vi "ShowSettingsDialog.vi"(10 "IMAQ Refnum in":refnum<k11>, 11 "Camera (in)":T1={"Framerate (Hz)"=100, "Exposure time (us)"=100, "Image size"={"Width"=1280, "Height"=1024}, "Number of buffers"=30}) -> (3 "Camera (out)":T1={"Framerate (Hz)"=100, "Exposure time (us)"=100, "Image size"={"Width"=1280, "Height"=1024}, "Number of buffers"=30})   [LabVIEW 2011]
uses:
  Main/Camera/GenericCameraConfigType.ctl
  Global_GenericIMAQCamera_HardwareConfig.vi
panel:
  in  "Set offsets to center frame":bool
  in  "Send serial cmd":bool
  out "Serial output":string
  in  "Serial input":string
  in  "Get current":bool
  in  "Camera":T1={"Framerate (Hz)"=100, "Exposure time (us)"=100, "Image size"={"Width"=1280, "Height"=1024}, "Number of buffers"=30}
  in  "Cancel":bool
  in  "Save":bool
  # "Dalsa Falcon2: Width needs to be a multiple of 128."
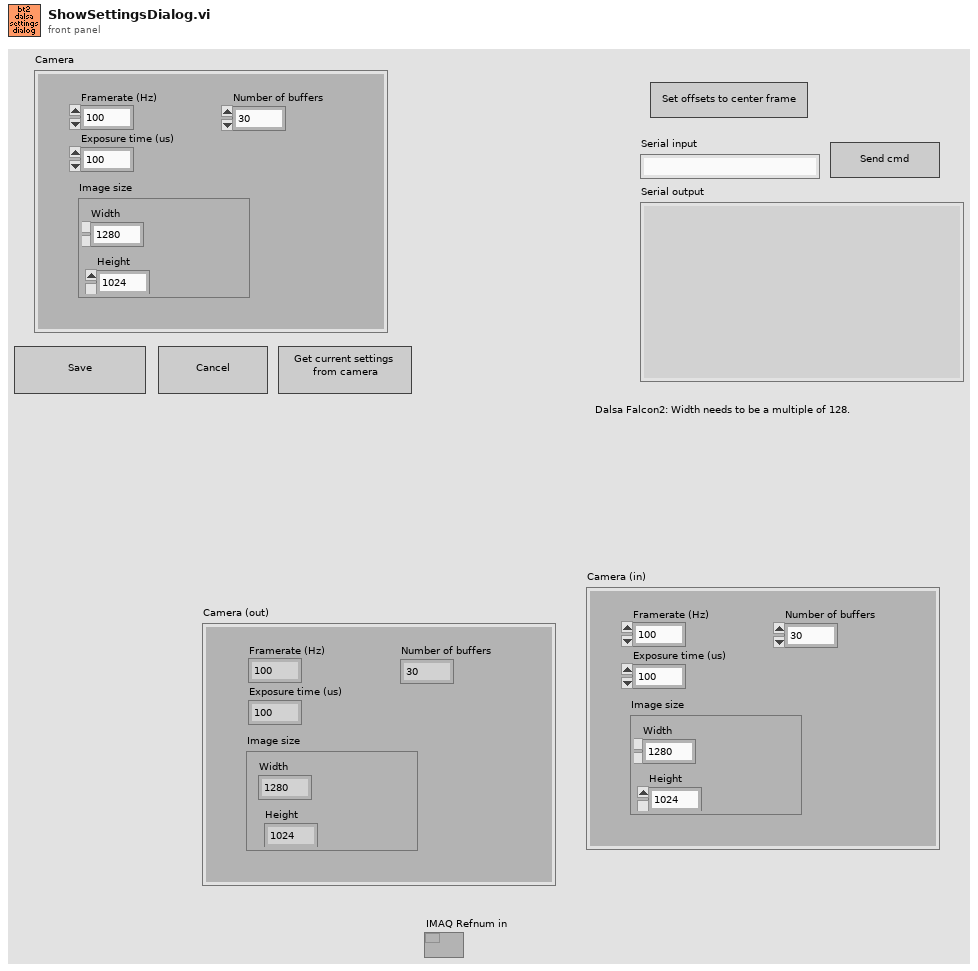
[diagram p1: front panel]
types:
  T1 = typedef "GenericCameraConfigType.ctl" = cluster{"Framerate (Hz)":i32, "Exposure time (us)":i32, "Image size":cluster{"Width":i32, "Height":i32}, "Number of buffers":i32}
  T2 = typedef "GenericIMAQHardwareConfig.ctl" = cluster{"Use serial commands directly":bool, "Frame rate set cmd":string, "Exposure time set cmd":string, "Frame rate get cmd":string, "Exposure time get cmd":string, "IMAQ Identifier":string, "Serial return skip chars":i32, "Set width/height":string, "Set offset xy":string, "Get width":string, "Get height":string, "Get offset X":string, "Get offset Y":string, "Full frame size":cluster{"width":i32, "height":i32}}
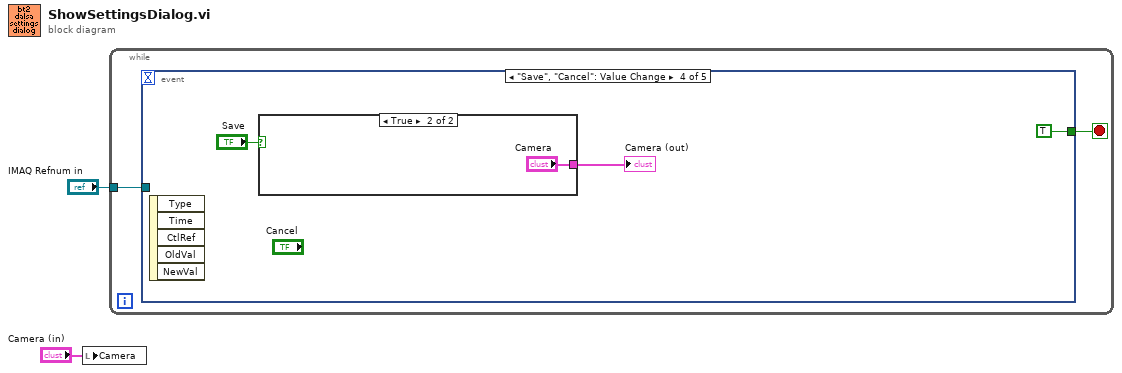
[diagram p0: block diagram]
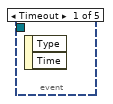
[diagram p2: hidden frame]
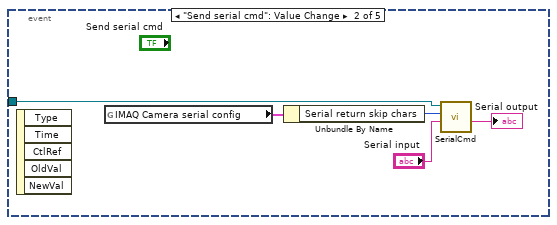
[diagram p3: hidden frame]
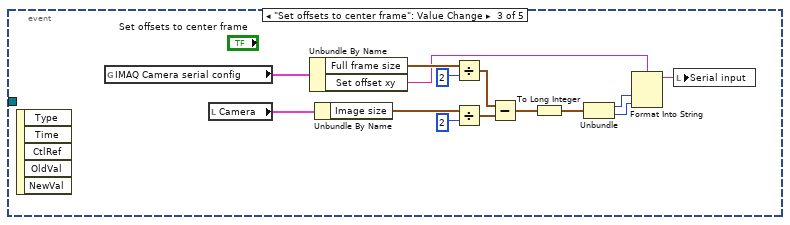
[diagram p4: hidden frame]
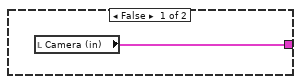
[diagram p5: hidden frame]
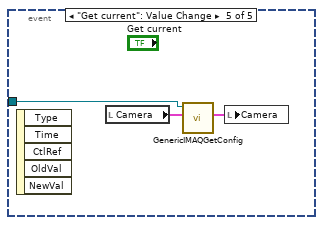
[diagram p6: hidden frame]
diagram:
  n1 = local write "Camera"("Camera (in)") -> ()
  n2 = while {
    tunnel: "IMAQ Refnum in" -> [w3]
    stop <- w4 stop-if-true
    n3 = event shown="[3] \"Save\", \"Cancel\": Value Change" {
      selector: _ -> [_ _ _ _ _]
      dyn-events: _ -> [_ _ _ _ _]
      timeout: _ -> [_ _ _ _ _]
      tunnel: [_ _ _ TRUE _] -> w4
      tunnel: w3 -> [_ w9 _ _ w31]
      event Timeout {
        n4 = event-data() -> ()  [unwired: 1 in, 2 out]
      }
      event "Send serial cmd": Value Change {
        n5 = event-data() -> ()  [unwired: 1 in, 5 out]
        n6 = global read "Global_GenericIMAQCamera_HardwareConfig.vi" "IMAQ Camera serial config"() -> (w6:T2)
        n7 = Unbundle By Name(w6) -> ("Serial return skip chars"=w5:i32)
        n8 = call "SerialCmd.vi"("command"="Serial input", "Return string skip chars (2)"=w5, "IMAQ Refnum in"=w9) -> ("String Read"=→"Serial output":string)  [unwired: 5 in, 3 out]
      }
      event "Set offsets to center frame": Value Change {
        n9 = event-data() -> ()  [unwired: 1 in, 5 out]
        n10 = global read "Global_GenericIMAQCamera_HardwareConfig.vi" "IMAQ Camera serial config"() -> (w22:T2)
        n11 = local read "Camera"() -> (w23:T1)
        n12 = Unbundle By Name(w22) -> ("Full frame size"=w21:cluster{"width":i32, "height":i32}, "Set offset xy"=w15:string)
        n13 = Unbundle By Name(w23) -> ("Image size"=w19:cluster{"Width":i32, "Height":i32})
        n14 = Divide(x=w21, y=2) -> (x/y=w17:cluster{"width":dbl, "height":dbl})
        n15 = Divide(x=w19, y=2) -> (x/y=w16:cluster{"Width":dbl, "Height":dbl})
        n16 = Subtract(x=w17, y=w16) -> (x-y=w12:cluster{dbl, dbl})
        n17 = To Long Integer(number=w12) -> (32bit integer=w11:cluster{i32, i32})
        n18 = Unbundle(w11) -> (w14:i32, w13:i32)
        n19 = Format Into String(format string=w15, w14, w13) -> (resulting string=w10:string)  [unwired: 2 in, 1 out]
        n20 = local write "Serial input"(w10) -> ()
      }
      event "Save", "Cancel": Value Change {
        n21 = event-data() -> ()  [unwired: 1 in, 5 out]
        n22 = case shown="True" "Save" {
          tunnel: [w27 "Camera"] -> w25
          frame False {
            n23 = local read "Camera (in)"() -> (w27:T1)
          }
          frame True {
          }
        }
        "Camera (out)" <- w25
      }
      event "Get current": Value Change {
        n24 = event-data() -> ()  [unwired: 1 in, 5 out]
        n25 = local read "Camera"() -> (w29:T1)
        n26 = call "GenericIMAQGetConfig.vi"("Camera (in)"=w29, "IMAQ Refnum in"=w31) -> ("Camera"=w30:T1)  [unwired: 8 in, 1 out]
        n27 = local write "Camera"(w30) -> ()
      }
    }
  }
